vi "MusclePower.vi"() -> ()   [LabVIEW 2016]
uses:
  <vilib>/express/express analysis/Spectral/Block/exnSpectralBlock spectral measurements power poly.vi
  <vilib>/express/express analysis/Spectral/Block/exnSpectralBlock spectral measurements power DDT.vi
  <vilib>/express/express analysis/Spectral/XNode/ExpressSpectralMeasurementsBlockNode.xnode
panel:
  out "?":dynamicdata(graph)
  out "data 2":dynamicdata(graph) caption="Raw Signal"
  in  "milliseconds to wait":u32
  in  "stop":bool
  out "?":dynamicdata(graph)
  out "data":dynamicdata(graph) caption="Processed Signal"
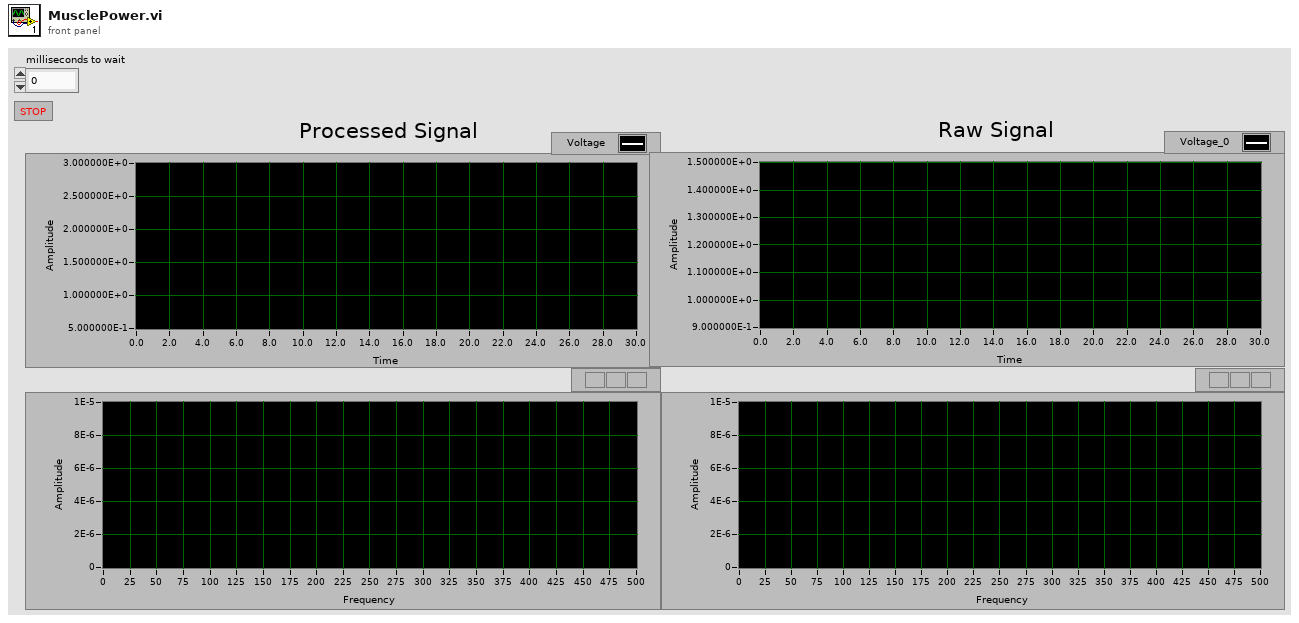
[diagram p1: front panel]
types:
  T1 = cluster{"averaging mode":u16, "weighting mode":u16, "number of averages":u32}
  T2 = cluster{"dB On (F)":bool, "unwrap phase (F)":bool, "convert to degree (F)":bool}
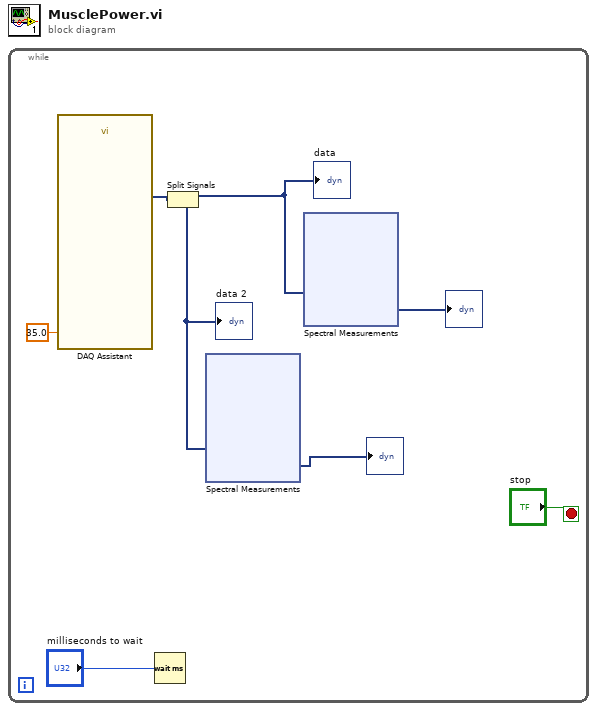
[diagram p0: block diagram]
diagram:
  n1 = while {
    stop <- "stop" stop-if-true
    n2 = call "DAQ Assistant"("timeout (s)"=35.0) -> ("data"=w6:dynamicdata)  [unwired: 16 in, 2 out]
    n3 = Wait (ms)(milliseconds to wait="milliseconds to wait") -> ()  [unwired: 1 out]
    n4 = Split Signals(w6) -> (w5:dynamicdata, w3:dynamicdata)  [unwired: 2 in]
    "data" <- w5
    "data 2" <- w3
    n5 = xnode "Spectral Measurements"("Signals"=w3) -> ("Power Spectrum"=→"?":dynamicdata)  [unwired: 1 in, 1 out]
    n6 = xnode "Spectral Measurements"("Signals"=w5) -> ("Power Spectrum"=→"?":dynamicdata)  [unwired: 1 in, 1 out]
  }
